vi "convertToTF.vi"(11 "Boolean":bool) -> (3 "Text":string)   [LabVIEW 2020]
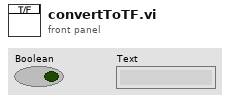
[diagram p1: front panel]
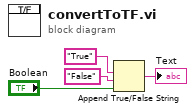
[diagram p0: block diagram]
diagram:
  n1 = Append True/False String(1:"Boolean", 2:"False" ("true string"), 3:"True" ("true string")) -> (0:→"Text":string)  [unwired: 1 in]
